vi "Fit_leak.vi"(6 "length":i32, 9 "start samples/time":i32, 11 "Waveform":waveform(dbl)) -> (2 "Leak (l/min)":dbl, 3 "Signal and fit":dbl[][](array[numeric]))   [LabVIEW 2016]
uses:
  <vilib>/Analysis/3filter.llb/Filter Passband Type.ctl
  <vilib>/Analysis/3filter.llb/Butterworth Filter (DBL).vi
  <vilib>/Analysis/NI_AALBase.lvlib
panel:
  out "Waveform 2":dbl[](graph)
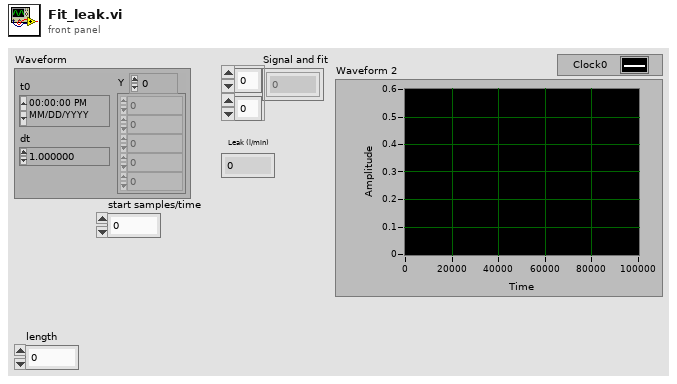
[diagram p1: front panel]
types:
  T1 = typedef "NI_AALBase.lvlib/Filter Passband Type.ctl" = enum32{"Lowpass", "Highpass", "Bandpass", "Bandstop"}
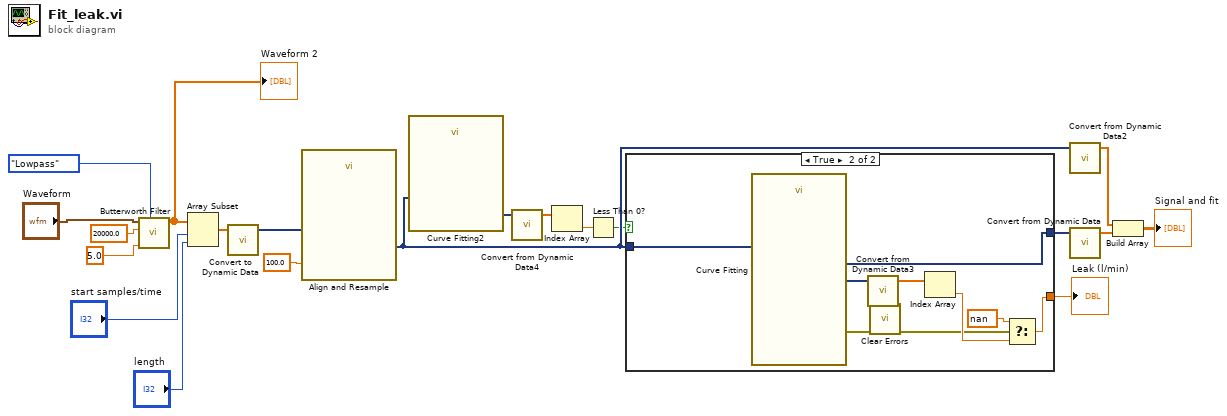
[diagram p0: block diagram]
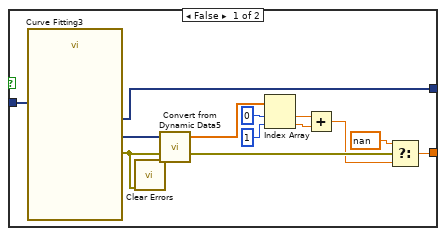
[diagram p2: hidden frame]
diagram:
  n1 = call-poly <vilib>:"Butterworth Filter.vi"("filter type"=Filter_Passband_Type."Lowpass", "low cutoff freq: fl"=5.0, "sampling freq: fs"=20000.0, "X"="Waveform") -> ("Filtered X"=w1:dbl[])  [unwired: 4 in, 1 out]
  "Waveform 2" <- w1
  n2 = Array Subset(array=w1, index="start samples/time", length="length") -> (w10:dbl[])
  n3 = call "Convert to Dynamic Data"("Array"=w10) -> ("Dynamic Data Type"=w3:dynamicdata)  [unwired: 3 in]
  n4 = call "Align and Resample"("dt"=100.0, "Signals"=w3) -> ("Resampled Signals"=w9:dynamicdata)  [unwired: 7 in, 2 out]
  n5 = call "Curve Fitting2"("Signals"=w9) -> ("slope"=w8:dynamicdata)  [unwired: 5 in, 5 out]
  n6 = call "Convert from Dynamic Data4"("Dynamic Data Type"=w8) -> ("Array"=w7:dbl[])  [unwired: 3 in]
  n7 = Index Array(array=w7) -> (element=w6:dbl)  [unwired: 1 in]
  n8 = Less Than 0?(x=w6) -> (x < 0?=w5:bool)
  n9 = case shown="True" w5 {
    tunnel: [w31 w41] -> w15
    tunnel: w9 -> [w32 w40]
    tunnel: [w21 w33] -> w4
    frame False {
      n10 = call "Curve Fitting3"("Signals"=w32) -> ("error out"=w24:errorcluster, "best fit"=w31:dynamicdata, "non-linear coefficients"=w30:dynamicdata)  [unwired: 6 in, 2 out]
      n11 = call <vilib>:"Clear Errors.vi"("error in (no error)"=w24) -> ()  [unwired: 5 in, 2 out]
      n12 = call "Convert from Dynamic Data5"("Dynamic Data Type"=w30) -> ("Array"=w27:dbl[])  [unwired: 3 in]
      n13 = Index Array(array=w27, index #1=0 ("index"), index #2=1 ("index")) -> (element #1=w26:dbl, element #2=w25:dbl)
      n14 = Add(x=w26, y=w25) -> (x+y=w23:dbl)
      n15 = Select(t=nan ("x+y"), s=w24, f=w23) -> (s? t:f=w21:dbl)
    }
    frame True {
      n16 = call "Curve Fitting"("Signals"=w40) -> ("error out"=w37:errorcluster, "best fit"=w41:dynamicdata, "non-linear coefficients"=w39:dynamicdata)  [unwired: 6 in, 2 out]
      n17 = call "Convert from Dynamic Data3"("Dynamic Data Type"=w39) -> ("Array"=w38:dbl[])  [unwired: 3 in]
      n18 = call <vilib>:"Clear Errors.vi"("error in (no error)"=w37) -> ("error out"=w34:errorcluster)  [unwired: 5 in, 1 out]
      n19 = Index Array(array=w38) -> (element=w35:dbl)  [unwired: 1 in]
      n20 = Select(t=nan ("x+y"), s=w34, f=w35) -> (s? t:f=w33:dbl)
    }
  }
  "Leak (l/min)" <- w4
  n21 = call "Convert from Dynamic Data2"("Dynamic Data Type"=w9) -> ("Array"=w18:dbl[])  [unwired: 3 in]
  n22 = call "Convert from Dynamic Data"("Dynamic Data Type"=w15) -> ("Array"=w16:dbl[])  [unwired: 3 in]
  n23 = Build Array(w18, w16) -> (→"Signal and fit":dbl[][])
